vi "Load Forbidden Package Names.vi"() -> (3 "Forbidden Packages":set{string}(c389))   [LabVIEW 2019, in "Project.Dependencies Finder.lvlib" / "Dependency Source_VIPM.lvclass"]
uses:
  Dependency Source_VIPM.lvclass
  Project.Dependencies Finder.lvlib
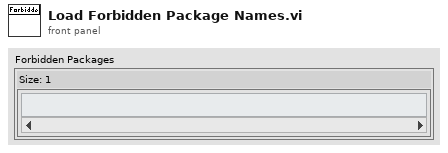
[diagram p1: front panel]
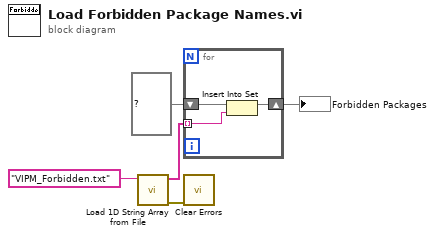
[diagram p0: block diagram]
diagram:
  n1 = call "Load 1D String Array from File.vi"("File name"="VIPM_Forbidden.txt") -> ("error out"=w1:errorcluster, "Loaded 1D String Array"=w2:string[])  [unwired: 9 in]
  n2 = for {
    shift-right: [w7] -> w3
    shift-left: set{string} {} ("set") -> [w8]
    tunnel: w2 -> [w6] mode=indexing
    n3 = Insert Into Set(10:w6, 11:w8) -> (3:w7:set{string})  [unwired: 1 out]
  }
  "Forbidden Packages" <- w3
  n4 = call <vilib>:"Clear Errors.vi"("error in (no error)"=w1) -> ()  [unwired: 5 in, 2 out]
